vi "Read.vi"(8 "error in":errorcluster, 11 "Serial Session in":refnum<class "Serial Session.lvclass">) -> (0 "error out":errorcluster, 2 "Data Out":string, 3 "Serial Session out":refnum<class "Serial Session.lvclass">)   [LabVIEW 2015, in "Serial Session.lvclass"]
doc: "Returns data from a serial device based on a asynchrnous read.\n\nHow this VI reads from the port is depending on how it is configured. If the read terminates on a character, then we simply request a read. If there is no termination charcater then we will wait for bytes based on the properties <b>Timeout (ms)</b> and <b>Loop Time (ms)</b>. In this latter case, we will read from the port based on checking the port regularly, based on the <b>Loop Time (ms)</b> property. The loop will complete after n = <b>Timeout (ms)/Loop Time (ms)</b> times or if there are no bytes on the port.\n\nThe output data string is trimmed to remove any leading or proceceding whitespace."
uses:
  Serial Session.lvclass
  Serial Session.lvclass/Serial Session.ctl
  <vilib>/Platform/TimedLoop/XDataNode/timing_clust.ctl
  <vilib>/Platform/TimedLoop/XDataNode/nitl_modes.ctl
  <vilib>/Platform/TimedLoop/XDataNode/wakeup.ctl
  <userlib>/_OpenG.lib/string/string.llb/Trim Whitespace (String)__ogtk.vi
  <vilib>/Platform/TimedLoop/XDataNode/XDataNode.xnode
  <vilib>/Platform/TimedLoop/XDataNode/XDNodeRunTimeDep.lvlib
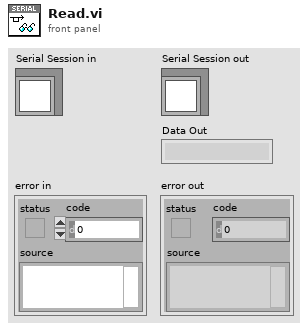
[diagram p1: front panel]
types:
  T1 = typedef "XDNodeRunTimeDep.lvlib/timing_clust.ctl" = cluster{"Expected End [f-1]":u64, "Actual End [f-1]":u64, "Finished Late? [f-1]":bool, "Expected End [i-1]":u64, "Actual End [i-1]":u64, "Finished Late? [i-1]":bool, "Expected Start [i]":u64, "Actual Start [i]":u64, "Expected Start [f]":u64, "Actual Start [f]":u64, "Source Name":string, "Structure Name":string, "Period":i64, "Deadline":i64, "Offset":i64, "Start":i64, "Priority":i32, "Timeout":i32, "Mode":T2, "Wakeup Reason":T3, "Error":errorcluster, "Source Type":string, "Secondary Source Type":string, "Global End Time":u64, "Global Start Time":u64, "Frame Duration":u64, "Iteration Duration":u64, "Assigned CPU":i32, "I/O Scan Engine Mode":u32}
  T2 = typedef "XDNodeRunTimeDep.lvlib/nitl_modes.ctl" = enum32{"No Change", "Process missed periods, maintain original phase", "Discard missed periods, maintain original phase", "Process missed periods, ignore original phase", "Discard missed periods, ignore original phase"}
  T3 = typedef "XDNodeRunTimeDep.lvlib/wakeup.ctl" = enum32{"Normal", "Aborted", "Asynchronous wakeup", "Timing source error", "Timed loop error", "Timeout"}
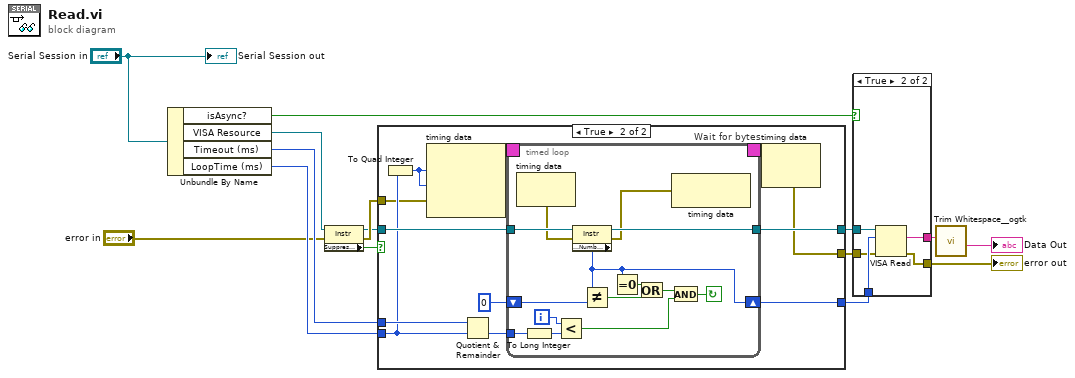
[diagram p0: block diagram]
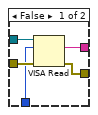
[diagram p2: hidden frame]
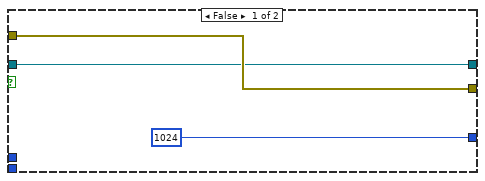
[diagram p3: hidden frame]
diagram:
  n1 = Unbundle By Name("Serial Session in") -> ("isAsync?"=w3:bool, "VISA Resource"=w14:refnum<visa-resource-name>, "Timeout (ms)"=w10:u32, "LoopTime (ms)"=w9:u32)
  n2 = property class="Instr"(reference=w14, error in="error in") -> (reference out=w11:refnum<visa-resource-name>, error out=w12:errorcluster, "Suppress End En"=w13:bool)
  n3 = case shown="True" w13 {
    tunnel: w11 -> [w17 w28]
    tunnel: [w17 w27] -> w8
    tunnel: [u32 1024 w26] -> w7
    tunnel: w10 -> [_ w25]
    tunnel: w9 -> [_ w24]
    tunnel: w12 -> [w18 w23]
    tunnel: [w18 w22] -> w6
    frame False {
    }
    frame True {
      n4 = To Quad Integer(1:w24) -> (0:w19:i64)
      n5 = node-c288(w19, w19, w23) -> (w30:T1)
      n6 = Quotient & Remainder(x=w25, y=w24) -> (floor(x/y)=w21:u32)  [unwired: 1 out]
      n7 = timed-loop "Wait for bytes" {
        tunnel: w28 -> [w44]
        tunnel: [w43] -> w27
        tunnel: w21 -> [w32]
        shift-right: [w35] -> w26
        shift-left: u32 0 -> [w36]
        timing: w30 -> [_]
        timing-out: [_] -> w29
        i -> [w42]
        stop <- w41 continue-if-true
        n8 = node-c288() -> (w34:errorcluster)  [unwired: 1 in]
        n9 = To Long Integer(number=w32) -> (32bit integer=w31:i32)
        n10 = Less?(x=w42, y=w31) -> (x < y?=w40:bool)
        n11 = property class="Instr"(reference=w44, error in=w34) -> (reference out=w43:refnum<visa-resource-name>, error out=w33:errorcluster, "Serial Settings:Number of Bytes at Serial Port"=w35:u32)
        n12 = Not Equal?(x=w35, y=w36) -> (x != y?=w39:bool)
        n13 = Equal To 0?(x=w35) -> (x = 0?=w38:bool)
        n14 = Or(x=w38, y=w39) -> (x .or. y?=w37:bool)
        n15 = And(x=w37, y=w40) -> (x .and. y?=w41:bool)
        n16 = node-c288(w33) -> ()  [unwired: 1 out]
      }
      n17 = node-c288(w29) -> (w22:errorcluster)
    }
  }
  n18 = case shown="True" w3 {
    tunnel: w8 -> [w61 w66]
    tunnel: w7 -> [w59 w65]
    tunnel: w6 -> [w60 w64]
    tunnel: [w57 w63] -> w4
    tunnel: [w58 w62] -> w2
    frame False {
      n19 = VISA Read(VISA resource name=w61, byte count=w59, error in (no error)=w60) -> (read buffer=w58:string, error out=w57:errorcluster)  [unwired: 2 out]
    }
    frame True {
      n20 = VISA Read(VISA resource name=w66, byte count=w65, error in (no error)=w64) -> (read buffer=w62:string, error out=w63:errorcluster)  [unwired: 2 out]
    }
  }
  "error out" <- w4
  n21 = call-poly <userlib>:"Trim Whitespace__ogtk.vi"("String in"=w2) -> ("String out"=→"Data Out":string)  [unwired: 6 in]
  "Serial Session out" <- "Serial Session in"
